vi "MainTestDemo.vi"() -> ()   [LabVIEW 2010]
uses:
  ROS/parsing/std_msgs/subs/parse_time_scalar.vi
  ROS/Code/SubVIs/_ROSDirection.ctl
panel:
  in  "Tab Control":T1(tab)
  out "Time":cluster{"secs":i32, "nsecs":i32}
  in  "Load Boxes":bool
  out "WorldProperties":T2
  out "link names":string[](array[string])
  out "Link Poses":T3(array[cluster]) {"Point"."y" format="%#_3f"}
  out "Link Twists":T4(array[cluster])
  out "link names 2":string[](array[string])
  out "Link Twists 2":T4(array[cluster])
  out "Link Poses 2":T3(array[cluster]) {"Point"."y" format="%#_3f"}
  in  "Twist 2":T5
  in  "Pose 2":T6 {"Point"."x" scale=-3.0..3.0}
  in  "Pose":T6 {"Point"."x" scale=-3.0..3.0}
  in  "Twist":T5
  in  "Boolean":bool
  in  "stop":bool
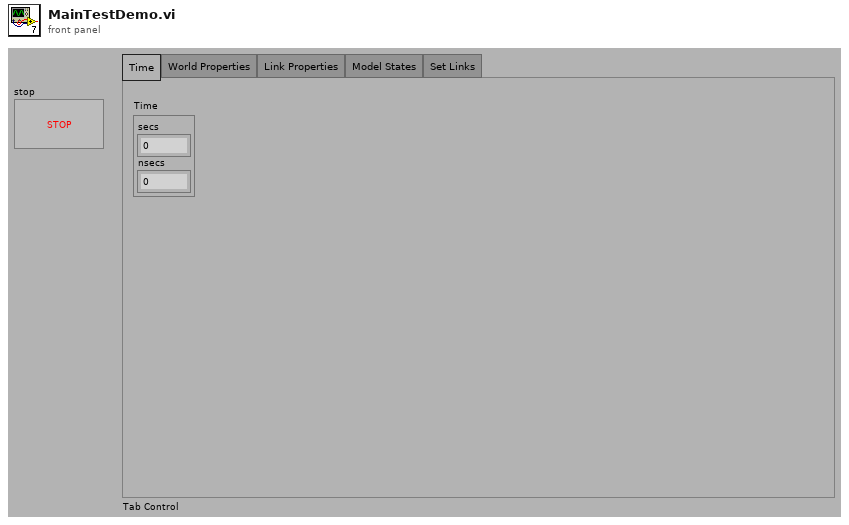
[diagram p1: front panel]
types:
  T1 = enum32{"Time", "World Properties", "Link Properties", "Model States", "Set Links"}
  T2 = cluster{"sim_time":dbl, "model_names":string[], "rendering enabled":bool, "success":bool, "status message":string}
  T3 = cluster{"Point":cluster{"x":dbl, "y":dbl, "z":dbl}, "Quaternion":cluster{"x":dbl, "y":dbl, "z":dbl, "w":dbl}}[]
  T4 = cluster{"Linear":cluster{"x":dbl, "y":dbl, "z":dbl}, "Angular":cluster{"x":dbl, "y":dbl, "z":dbl}}[]
  T5 = cluster{"Linear":cluster{"x":dbl, "y":dbl, "z":dbl}, "Angular":cluster{"x":dbl, "y":dbl, "z":dbl}}
  T6 = cluster{"Point":cluster{"x":dbl, "y":dbl, "z":dbl}, "Quaternion":cluster{"x":dbl, "y":dbl, "z":dbl, "w":dbl}}
  T7 = typedef "_ROSDirection.ctl" = enum16{"Node", "Publisher", "Subscriber", "Service Client"}
  T8 = cluster{"Topic":string, "Type":string, "Action":T7, "Update (ms)":u16, "write queue":u16}
  T9 = typedef "_ROSControl.ctl" = cluster{"topic port":u16, "Node":string, "topic":string, "type":string, "node port":u32, "error ":errorcluster, "Direction":T7, "APIs":string[], "Update (ms)":u16, "write queue":u16}
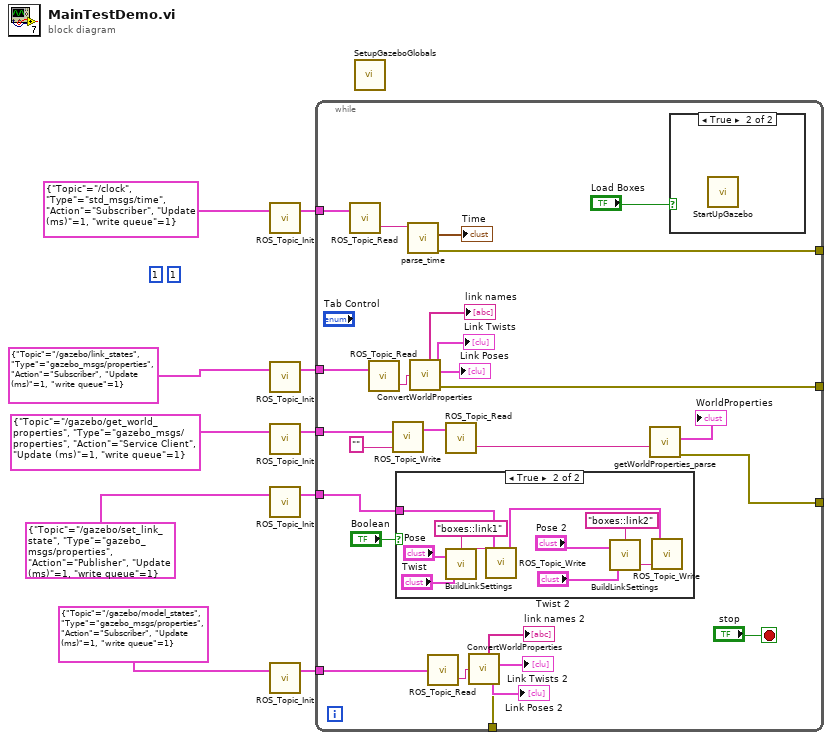
[diagram p0: block diagram]
diagram:
  (unwired) u16 1 ("write queue")
  (unwired) u16 1 ("Update (ms)")
  n1 = call "ROS_Topic_Init.vi"("Definitions"=T8 {"Topic"="/clock", "Type"="std_msgs/time", "Action"=enum."Subscriber", "Update (ms)"=1, "write queue"=1} ("element")) -> ("ROS out"=w10:T9)  [unwired: 2 in]
  n2 = call "ROS_Topic_Init.vi"("Definitions"=T8 {"Topic"="/gazebo/link_states", "Type"="gazebo_msgs/properties", "Action"=enum."Subscriber", "Update (ms)"=1, "write queue"=1} ("element")) -> ("ROS out"=w8:T9)  [unwired: 2 in]
  n3 = call "ROS_Topic_Init.vi"("Definitions"=T8 {"Topic"="/gazebo/get_world_properties", "Type"="gazebo_msgs/properties", "Action"=enum."Service Client", "Update (ms)"=1, "write queue"=1} ("element")) -> ("ROS out"=w9:T9)  [unwired: 2 in]
  n4 = call "ROS_Topic_Init.vi"("Definitions"=T8 {"Topic"="/gazebo/set_link_state", "Type"="gazebo_msgs/properties", "Action"=enum."Publisher", "Update (ms)"=1, "write queue"=1} ("element")) -> ("ROS out"=w7:T9)  [unwired: 2 in]
  n5 = call "ROS_Topic_Init.vi"("Definitions"=T8 {"Topic"="/gazebo/model_states", "Type"="gazebo_msgs/properties", "Action"=enum."Subscriber", "Update (ms)"=1, "write queue"=1} ("element")) -> ("ROS out"=w6:T9)  [unwired: 2 in]
  n6 = while {
    tunnel: w10 -> [w36]
    tunnel: w9 -> [w35]
    tunnel: w8 -> [w34]
    tunnel: [w27] -> _
    tunnel: [w26] -> _
    tunnel: w7 -> [w23]
    tunnel: [w22] -> _
    tunnel: w6 -> [w14]
    tunnel: [w13] -> _
    stop <- "stop" stop-if-true
    n7 = call "ROS_Topic_Read.vi"("ROS in"=w36) -> ("Reply"=w31:string)  [unwired: 1 in, 1 out]
    n8 = call "ROS_Topic_Read.vi"("ROS in"=w34) -> ("Reply"=w24:string)  [unwired: 1 in, 1 out]
    n9 = call "ROS_Topic_Write.vi"("Msg in"="", "ROS in"=w35) -> ("ROS out"=w33:T9)  [unwired: 2 in]
    n10 = case shown="True" "Boolean" {
      tunnel: w23 -> [_ w46]
      frame False {
      }
      frame True {
        n11 = call "BuildLinkSettings.vi"("Twist"="Twist", "Pose"="Pose", "link to move"="boxes::link1") -> ("msg out"=w45:string)  [unwired: 1 in]
        n12 = call "ROS_Topic_Write.vi"("Msg in"=w45, "ROS in"=w46) -> ("ROS out"=w38:T9)  [unwired: 2 in]
        n13 = call "BuildLinkSettings.vi"("Twist"="Twist 2", "Pose"="Pose 2", "link to move"="boxes::link2") -> ("msg out"=w37:string)  [unwired: 1 in]
        n14 = call "ROS_Topic_Write.vi"("Msg in"=w37, "ROS in"=w38) -> ()  [unwired: 2 in, 1 out]
      }
    }
    n15 = call-poly "parse_time.vi"("msg in"=w31) -> ("error out"=w27:errorcluster, "Time"=→"Time":cluster{"secs":i32, "nsecs":i32})  [unwired: 4 in, 1 out]
    n16 = call "ConvertWorldProperties.vi"("Reply"=w24) -> ("Poses"=→"Link Poses":T3, "Twists"=→"Link Twists":T4, "error out"=w22:errorcluster, "names"=→"link names":string[])  [unwired: 1 in]
    n17 = call "ROS_Topic_Read.vi"("ROS in"=w14) -> ("Reply"=w16:string)  [unwired: 1 in, 1 out]
    n18 = call "ROS_Topic_Read.vi"("ROS in"=w33) -> ("Reply"=w32:string)  [unwired: 1 in, 1 out]
    n19 = call "ConvertWorldProperties.vi"("Reply"=w16) -> ("Poses"=→"Link Poses 2":T3, "Twists"=→"Link Twists 2":T4, "error out"=w13:errorcluster, "names"=→"link names 2":string[])  [unwired: 1 in]
    n20 = call "getWorldProperties_parse.vi"("msg in"=w32) -> ("error out"=w26:errorcluster, "WorldProperties"=→"WorldProperties":T2)  [unwired: 8 in, 1 out]
    n21 = case shown="True" "Load Boxes" {
      frame False {
      }
      frame True {
        n22 = call "StartUpGazebo.vi"() -> ()  [unwired: 12 in]
      }
    }
  }
  n23 = call "SetupGazeboGlobals.vi"() -> ()  [unwired: 4 in]
